vi "m10.wfg.01DC.vi"(1 "Param 0":dbl=1000.0, 2 "Param 1":dbl, 3 "Param 2":dbl, 4 "Param 3":dbl, 5 "error in (no error)":errorcluster, 8 "Waveform Properties":T1={"Fs (Hz)"=20000.0, "Amplitude (V)"=5.0, "Ramp (s)"=0.02, "Duration (s)"=0.1} {"Ramp (s)" min=0.0; "Fs (Hz)" min=0.0}) -> (14 "Waveform Out":waveform(dbl), 19 "error out":errorcluster)   [LabVIEW 2013]
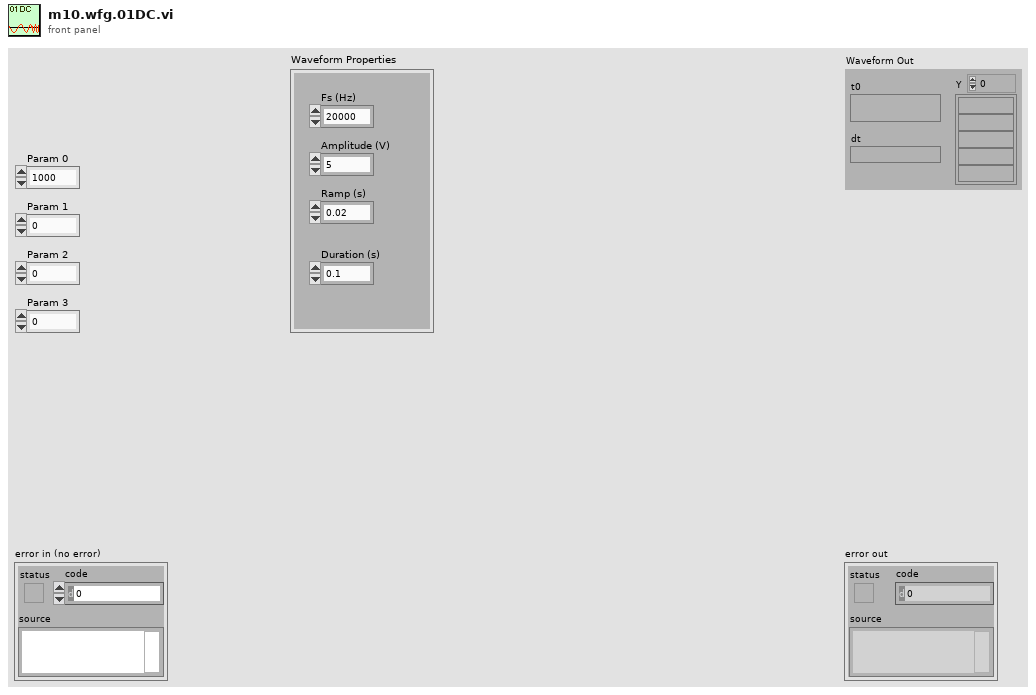
[diagram p1: front panel]
types:
  T1 = cluster{"Fs (Hz)":dbl, "Amplitude (V)":dbl, "Ramp (s)":dbl, "Duration (s)":dbl}
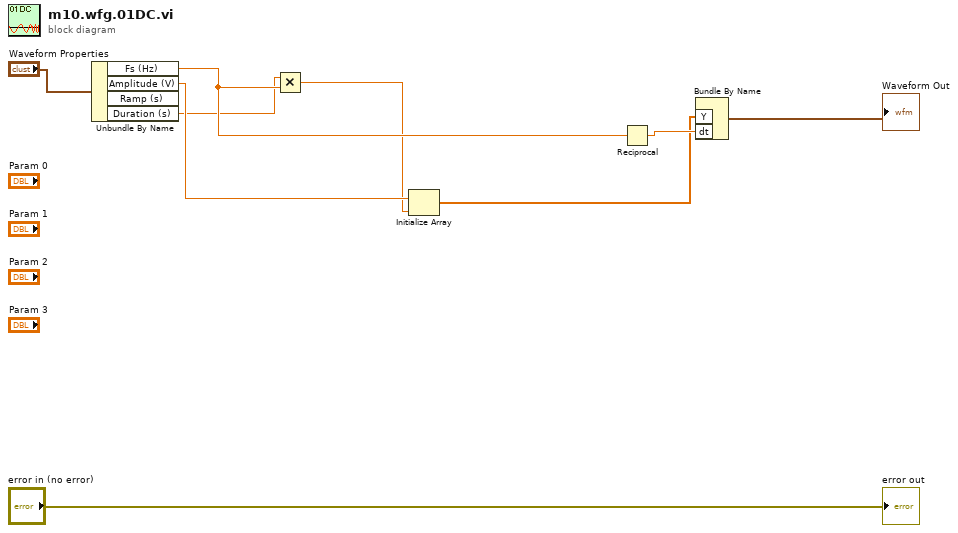
[diagram p0: block diagram]
diagram:
  n1 = Unbundle By Name("Waveform Properties") -> ("Fs (Hz)"=w6:dbl, "Amplitude (V)"=w5:dbl, "Duration (s)"=w1:dbl)  [unwired: 1 out]
  n2 = Multiply(x=w1, y=w6) -> (x*y=w4:dbl)
  n3 = Initialize Array(w5, w4) -> (w3:dbl[])
  n4 = Reciprocal(x=w6) -> (1/x=w8:dbl)
  n5 = Bundle By Name("Y"=w3, "dt"=w8) -> (→"Waveform Out":waveform(dbl))  [unwired: 1 in]
  "error out" <- "error in (no error)"
